vi "monitorFileSize.vi"(8 "error in (no error)":errorcluster, 11 "Logger in":refnum<class "Logger.lvclass">) -> (0 "error out":errorcluster, 3 "Logger out":refnum<class "Logger.lvclass">)   [LabVIEW 2013, in "Logger.lvclass"]
uses:
  Logger.lvclass
  Logger.lvclass/Logger.ctl
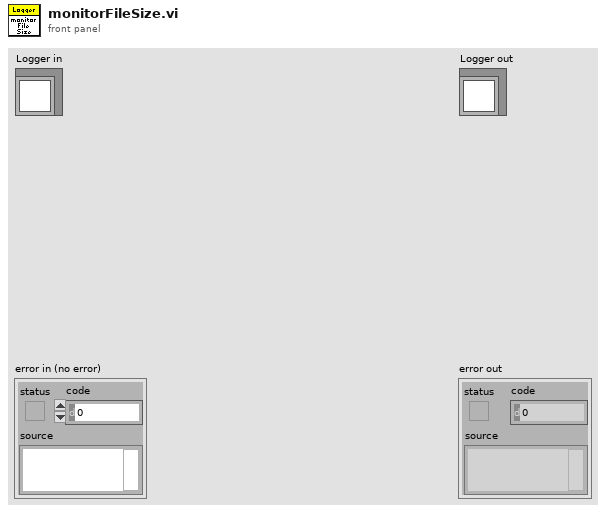
[diagram p1: front panel]
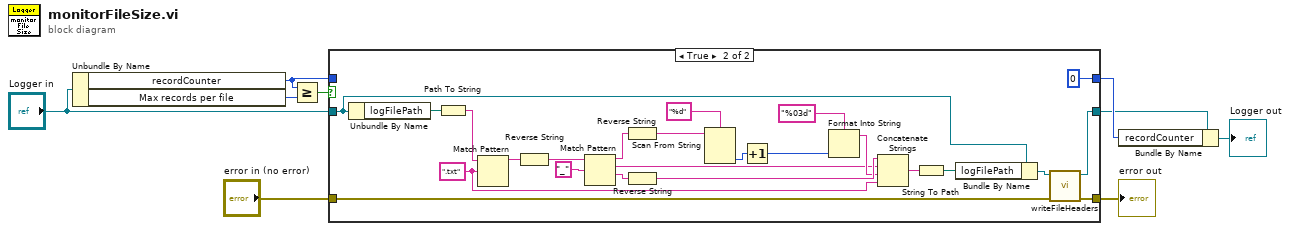
[diagram p0: block diagram]
diagram:
  n1 = Unbundle By Name("Logger in") -> ("recordCounter"=w1:u32, "Max records per file"=w7:u32)
  n2 = Greater Or Equal?(x=w1, y=w7) -> (x >= y?=w6:bool)
  n3 = case shown="True" w6 {
    tunnel: w1 -> [w10 _]
    tunnel: [w10 u32 0] -> w9
    tunnel: "Logger in" -> [w12 w23]
    tunnel: [w12 w15] -> w8
    tunnel: [w11 w14] -> w3
    tunnel: "error in (no error)" -> [w11 w13]
    frame False {
    }
    frame True {
      w24 = ".txt" ("regular expression")
      n4 = Unbundle By Name(w23) -> ("logFilePath"=w22:path)
      n5 = Path To String(path=w22) -> (string=w35:string)
      n6 = Match Pattern(string=w35, regular expression=w24) -> (before substring=w34:string)  [unwired: 1 in, 3 out]
      n7 = Reverse String(1:w34) -> (0:w33:string)
      n8 = Match Pattern(string=w33, regular expression="_") -> (before substring=w30:string, match substring=w18:string, after substring=w28:string)  [unwired: 1 in, 1 out]
      n9 = Reverse String(1:w30) -> (0:w17:string)
      n10 = Reverse String(1:w28) -> (0:w26:string)
      n11 = Scan From String(format string="%d", input string=w17) -> (output 1=w29:i32)  [unwired: 3 in, 3 out]
      n12 = Increment(x=w29) -> (x+1=w27:i32)
      n13 = Format Into String(format string="%03d", w27) -> (resulting string=w25:string)  [unwired: 2 in, 1 out]
      n14 = Concatenate Strings(w26, w18, w25, w24) -> (w21:string)
      n15 = String To Path(string=w21) -> (path=w20:path)
      n16 = Bundle By Name(cluster=w23, "logFilePath"=w20) -> (w16:refnum<class "Logger.lvclass">)
      n17 = call "writeFileHeaders.vi"("error in (no error)"=w13, "Logger in"=w16) -> ("error out"=w14:errorcluster, "Logger out"=w15:refnum<class "Logger.lvclass">)  [unwired: 8 in]
    }
  }
  "error out" <- w3
  n18 = Bundle By Name(cluster=w8, "recordCounter"=w9) -> (→"Logger out":refnum<class "Logger.lvclass">)
